vi "Create Generic Log Message.vi"(6 "Level":T1, 7 "Logger Name":string, 8 "error in (no error)":errorcluster, 10 "Message":string, 11 "Call Chain":string[](array[string])) -> (0 "error out":errorcluster)   [LabVIEW 2020, in "Global_logger.lvlib"]
uses:
  Global_logger.lvlib
  Levels.ctl
  Event.ctl
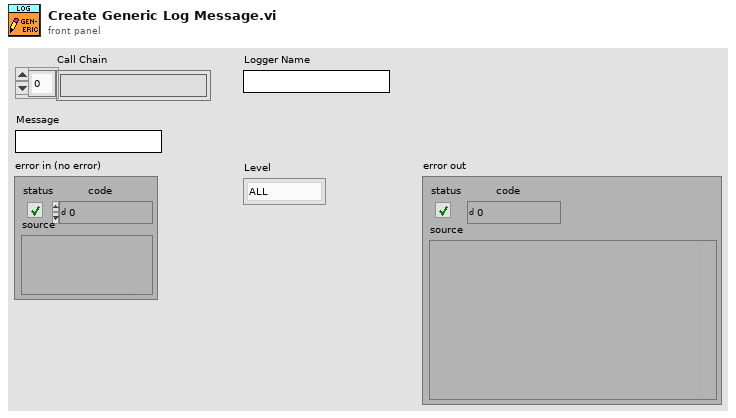
[diagram p1: front panel]
types:
  T1 = typedef "Global_logger.lvlib/Levels.ctl" = enum16{"ALL", "TRACE", "DEBUG", "INFO", "WARN", "ERROR", "FATAL", "OFF"}
  T2 = typedef "Global_logger.lvlib/Event.ctl" = cluster{"Logger Name":string, "Time Stamp":timestamp, "Level":T1, "Source VI":string, "Message":string, "Source App":string}
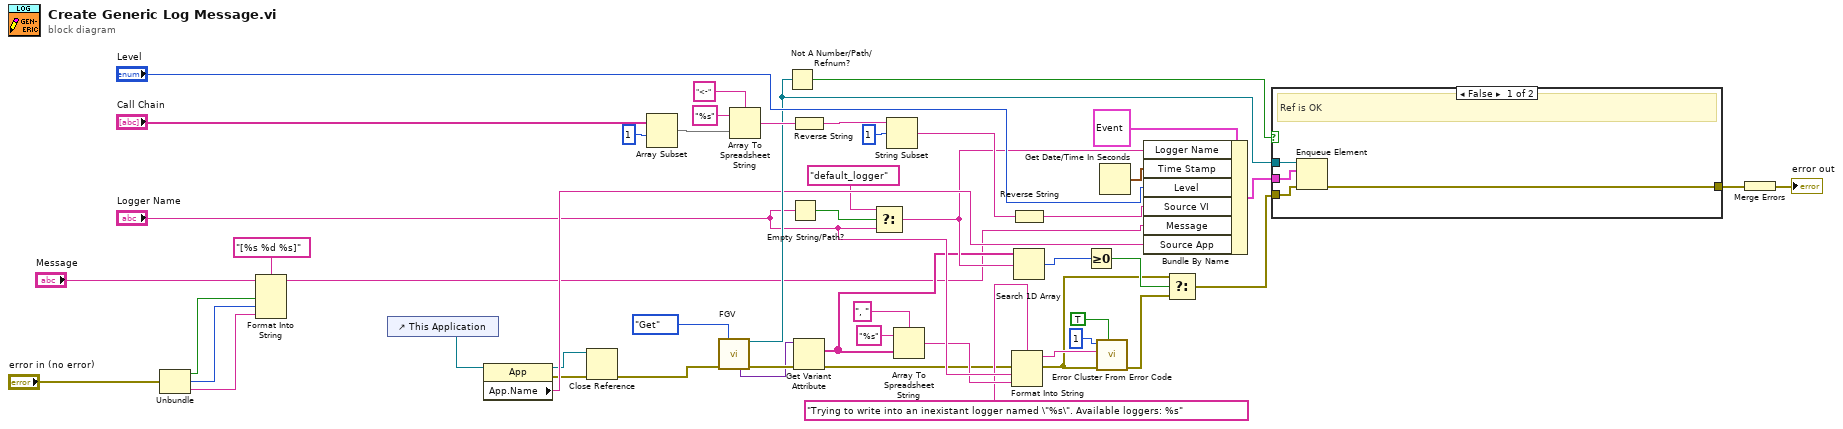
[diagram p0: block diagram]
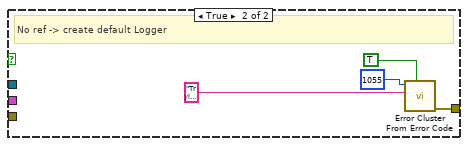
[diagram p2: hidden frame]
diagram:
  n1 = Unbundle("error in (no error)") -> ("status"=w4:bool, "code"=w3:i32, "source"=w2:string)
  n2 = Format Into String(format string="[%s %d %s]", initial string="Message", w4, w3, w2) -> (resulting string=w6:string)  [unwired: 1 in, 1 out]
  n3 = control-ref of="This Application"() -> (w29:refnum<vi>)
  n4 = property class="App"(reference=w29) -> (reference out=w27:refnum<vi>, error out=w30:errorcluster, "App.Name"=w31:string)  [unwired: 1 in]
  n5 = Close Reference(reference=w27, error in (no error)=w30) -> (error out=w28:errorcluster)
  n6 = Array Subset(array="Call Chain", index=1) -> (w36:string[])  [unwired: 1 in]
  n7 = call "FGV.vi"("Action"=enum16{"Get", "Set"}."Get", "error in (no error)"=w28) -> ("queue out"=w33:refnum<queue>, "All Named Loggers"=w23:variant, "error out"=w24:errorcluster)  [unwired: 8 in, 3 out]
  n8 = Array To Spreadsheet String(delimiter (Tab)="<-", array=w36, 3:"%s" ("format string")) -> (spreadsheet string=w42:string)
  n9 = Not A Number/Path/Refnum?(number/path/refnum=w33) -> (NaN/Path/Refnum?=w32:bool)
  n10 = Empty String/Path?(string/path="Logger Name") -> (empty?=w26:bool)
  n11 = Reverse String(1:w42) -> (0:w41:string)
  n12 = Get Variant Attribute(Variant=w23, error in=w24) -> (names=w18:string[], error out=w13:errorcluster)  [unwired: 2 in, 2 out]
  n13 = Select(t="default_logger", s=w26, f="Logger Name") -> (s? t:f=w22:string)
  n14 = String Subset(string=w41, offset (0)=1) -> (substring=w39:string)  [unwired: 1 in]
  n15 = Array To Spreadsheet String(delimiter (Tab)=", ", array=w18, 3:"%s" ("format string")) -> (spreadsheet string=w15:string)
  n16 = Format Into String(format string="Trying to write into an inexistant logger named \"%s\". Available loggers: %s", error in=w13, "Logger Name", w15) -> (resulting string=w12:string, error out=w8:errorcluster)  [unwired: 1 in]
  n17 = Reverse String(1:w39) -> (0:w38:string)
  n18 = Search 1D Array(1D array=w18, element=w22) -> (index of element=w21:i32)  [unwired: 1 in]
  n19 = Greater Or Equal To 0?(x=w21) -> (x >= 0?=w10:bool)
  n20 = call <vilib>:"Error Cluster From Error Code.vi"("show call chain? (False)"=TRUE, "error in (no error)"=w8, "error message (\"\")"=w12, "error code (0)"=1) -> ("error out"=w9:errorcluster)  [unwired: 5 in]
  n21 = Get Date/Time In Seconds() -> (seconds since 1Jan1904=w49:timestamp)
  n22 = Bundle By Name(cluster=T2 {"Logger Name"="", "Time Stamp"=timestamp(0 s since 1904-01-01), "Level"=enum."ALL", "Source VI"="", "Message"="", "Source App"=""} ("element"), "Logger Name"=w22, "Time Stamp"=w49, "Level"="Level", "Source VI"=w38, "Message"=w6, "Source App"=w31) -> (w48:T2)
  n23 = Select(t=w8, s=w10, f=w9) -> (s? t:f=w7:errorcluster)
  n24 = case shown="False" w32 {
    tunnel: w48 -> [w55 _]
    tunnel: [w54 w57] -> w35
    tunnel: w33 -> [w53 _]
    tunnel: w7 -> [w52 _]
    frame False {
      # "Ref is OK"
      n25 = Enqueue Element(queue=w53, element=w55, error in (no error)=w52) -> (error out=w54:errorcluster)  [unwired: 1 in, 2 out]
    }
    frame True {
      # "No ref -> create default Logger"
      n26 = call <vilib>:"Error Cluster From Error Code.vi"("show call chain? (False)"=TRUE, "error message (\"\")"="Trying to write a log record before any logger was created" ("error message (\"\")"), "error code (0)"=1055) -> ("error out"=w57:errorcluster)  [unwired: 6 in]
    }
  }
  n27 = Merge Errors(w35) -> (→"error out":errorcluster)
